vi "Error Loop Data.vi"(7 "Data Functions":T2, 8 "error in (no error)":errorcluster) -> (0 "error out":errorcluster, 3 "Error Data Reference":T1)   [LabVIEW 2016, in "System.lvlib"]
uses:
  System.lvlib
  Controls/Control_Data Functions.ctl
  Controls/Control_Variant Data Reference.ctl
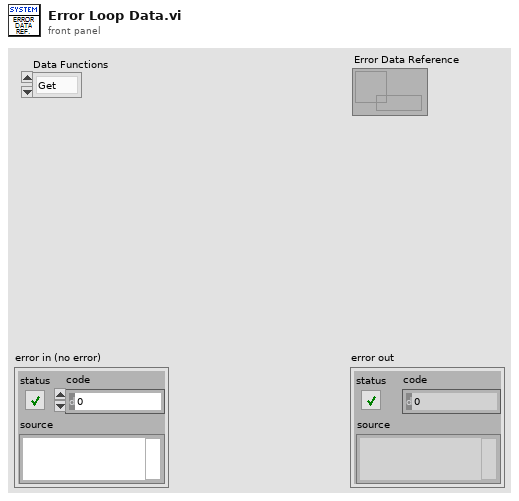
[diagram p1: front panel]
types:
  T1 = typedef "System.lvlib/Control_Variant Data Reference.ctl" = refnum<data-value>
  T2 = typedef "System.lvlib/Control_Data Functions.ctl" = enum16{"Get", "Set", "Release"}
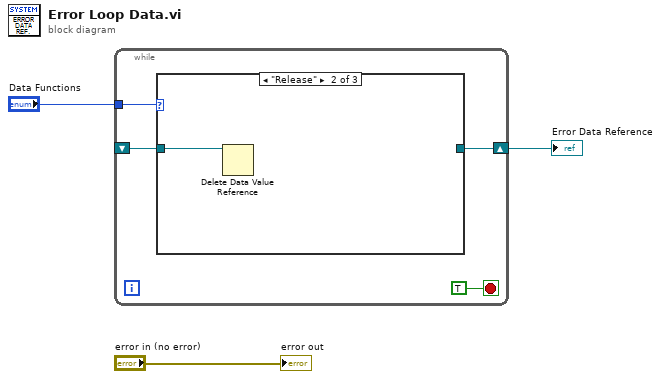
[diagram p0: block diagram]
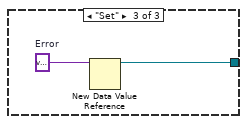
[diagram p3: hidden frame]
diagram:
  n1 = while {
    tunnel: "Data Functions" -> [w6]
    shift-right: [w5] -> w2
    shift-left: _ -> [w4]
    stop <- TRUE stop-if-true
    n2 = case shown="\"Release\"" w6 {
      tunnel: [w8 _ w11] -> w5
      tunnel: w4 -> [w8 w9 _]
      frame "Get", Default {
      }
      frame "Release" {
        n3 = Delete Data Value Reference(data value reference=w9) -> ()  [unwired: 1 in, 2 out]
      }
      frame "Set" {
        w10 = variant  # Error
        n4 = New Data Value Reference(data value=w10) -> (data value reference=w11:refnum<data-value>)  [unwired: 1 in, 1 out]
      }
    }
  }
  "Error Data Reference" <- w2
  "error out" <- "error in (no error)"
